vi "Gate Delay Calc.vi"(3 "Percent":dbl, 4 "Frequency":dbl[unit], 5 "gatedelayoffsetB":dbl[unit], 6 "gatedelayoffsetA":dbl[unit]) -> (0 "Gate Width":dbl[unit], 1 "Gate B Delay":dbl[unit], 2 "Gate A Delay":dbl[unit])   [LabVIEW 2012, in "Photon Counter SR400.lvclass"]
uses:
  Photon Counter SR400.lvclass
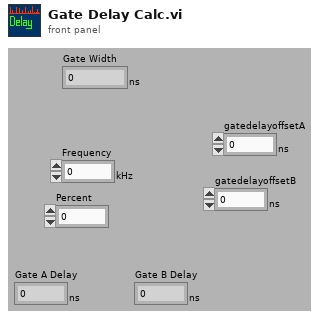
[diagram p1: front panel]
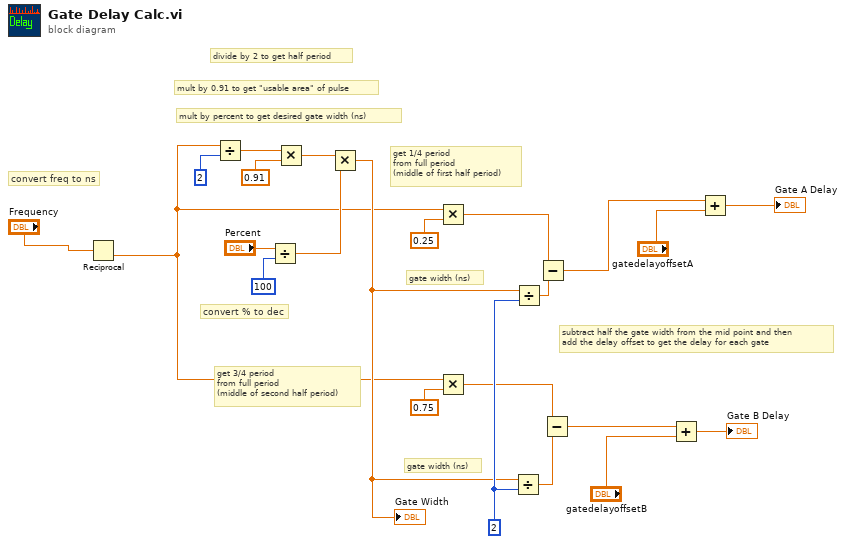
[diagram p0: block diagram]
diagram:
  w23 = 2
  # "subtract half the gate width from the mid point and then\nadd the delay offset to get the delay for each gate"
  # "gate width (ns)"
  # "gate width (ns)"
  # "mult by percent to get desired gate width (ns)"
  # "get 3/4 period\nfrom full period\n(middle of second half period)"
  # "get 1/4 period\nfrom full period\n(middle of first half period)"
  # "convert % to dec"
  # "mult by 0.91 to get \"usable area\" of pulse"
  # "divide by 2 to get half period"
  # "convert freq to ns"
  n1 = Reciprocal(x="Frequency") -> (1/x=w1:dbl[unit])
  n2 = Divide(x=w1, y=2) -> (x/y=w15:dbl[unit])
  n3 = Divide(x="Percent", y=100) -> (x/y=w4:dbl)
  n4 = Multiply(x=w15, y=0.91) -> (x*y=w13:dbl[unit])
  n5 = Multiply(x=w13, y=w4) -> (x*y=w11:dbl[unit])
  "Gate Width" <- w11
  n6 = Multiply(x=w1, y=0.25) -> (x*y=w19:dbl[unit])
  n7 = Multiply(x=w1, y=0.75) -> (x*y=w18:dbl[unit])
  n8 = Divide(x=w11, y=w23) -> (x/y=w22:dbl[unit])
  n9 = Divide(x=w11, y=w23) -> (x/y=w21:dbl[unit])
  n10 = Subtract(x=w19, y=w21) -> (x-y=w10:dbl[unit])
  n11 = Subtract(x=w18, y=w22) -> (x-y=w7:dbl[unit])
  n12 = Add(x=w7, y="gatedelayoffsetB") -> (x+y=→"Gate B Delay":dbl[unit])
  n13 = Add(x=w10, y="gatedelayoffsetA") -> (x+y=→"Gate A Delay":dbl[unit])
